vi "AngleSpect.vi"(3 "Angle In":dbl, 4 "Angle Tolerance":dbl, 5 "Angle  Spect":dbl) -> (0 "Angle Color":u32, 2 "Angle OK":bool)   [LabVIEW 2017]
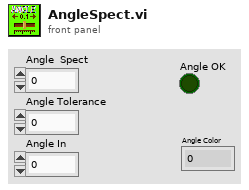
[diagram p1: front panel]
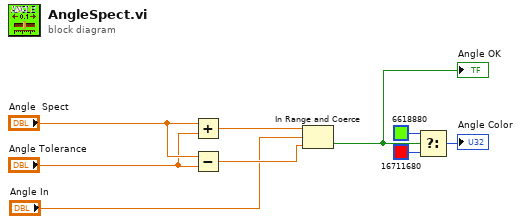
[diagram p0: block diagram]
diagram:
  n1 = Add(x="Angle  Spect", y="Angle Tolerance") -> (x+y=w7:dbl)
  n2 = Subtract(x="Angle  Spect", y="Angle Tolerance") -> (x-y=w6:dbl)
  n3 = In Range and Coerce(upper limit=w7, x="Angle In", lower limit=w6) -> (In Range?=w4:bool)  [unwired: 1 out]
  "Angle OK" <- w4
  n4 = Select(t=u32 6618880, s=w4, f=u32 16711680) -> (s? t:f=→"Angle Color":u32)
